vi "Config.vi"() -> ()   [LabVIEW 2020]
uses:
  Global_Variable/Global.vi
  Global_Variable/A180648.vi
  <vilib>/Utility/config.llb/NI_LVConfig.lvlib
  Libraries/S7/S7.lvlib
panel:
  in  "判定框参数":string[][](table)=[["mm"], ["KN"], ["mm"], ["KN"]]
  in  "结果判定参数":string[][](table)=[["mm"], ["KN"], ["KN"], ["KN"], [""], [""], [""], [""], [""], [""], [""], [""]]
  in  "坐标轴参数":string[][](table)=[[""], ["°/S"], ["°"], ["Nm"]]
  in  "试验项目":cluster{"拉轴":bool, "卡簧":bool}
  in  "产品型号":string(combo)
  in  "删除":bool
  in  "确定":bool
  in  "添加":bool
  in  "退出":bool
  in  "更新":bool
  # "上管柱上转向轴合成"
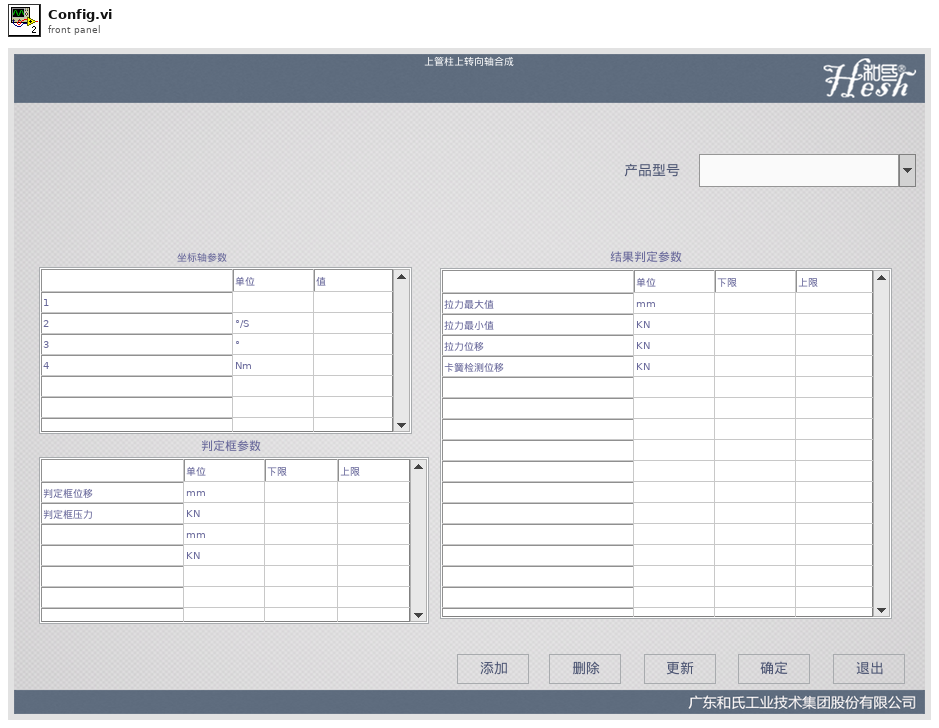
[diagram p1: front panel]
types:
  T1 = typedef "NI_LVConfig.lvlib/Config Data RefNum.ctl" = refnum<k1>
  T2 = cluster{"[0]":cluster{string, dbl, dbl}, "[1]":cluster{string, dbl, dbl}}
  T3 = cluster{"1位移":cluster{"单位":string, "下限":dbl, "上限":dbl}, "1压力":cluster{"单位":string, "下限":dbl, "上限":dbl}}
  T4 = cluster{"[0]":cluster{string, dbl, dbl}, "[1]":cluster{string, dbl, dbl}, "[2]":cluster{string, dbl, dbl}}
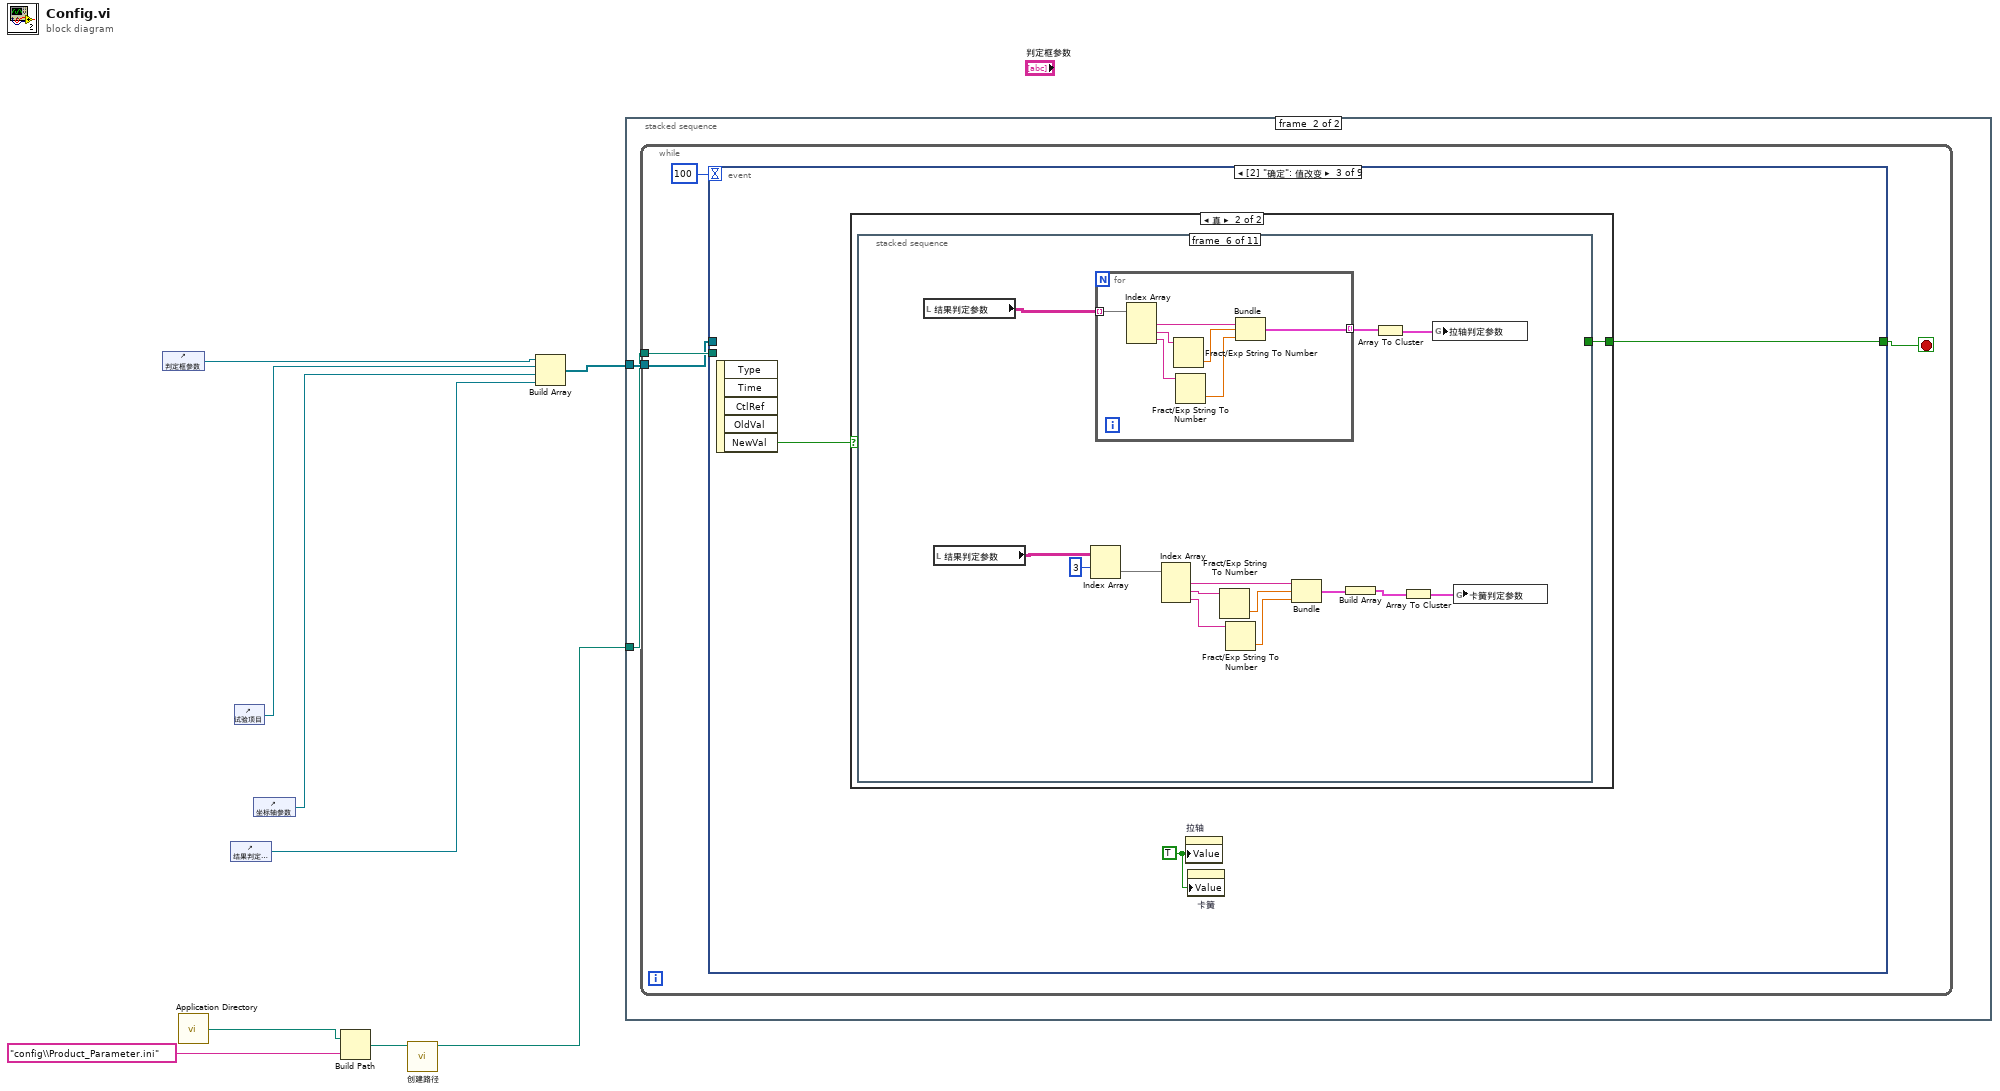
[diagram p0: block diagram]
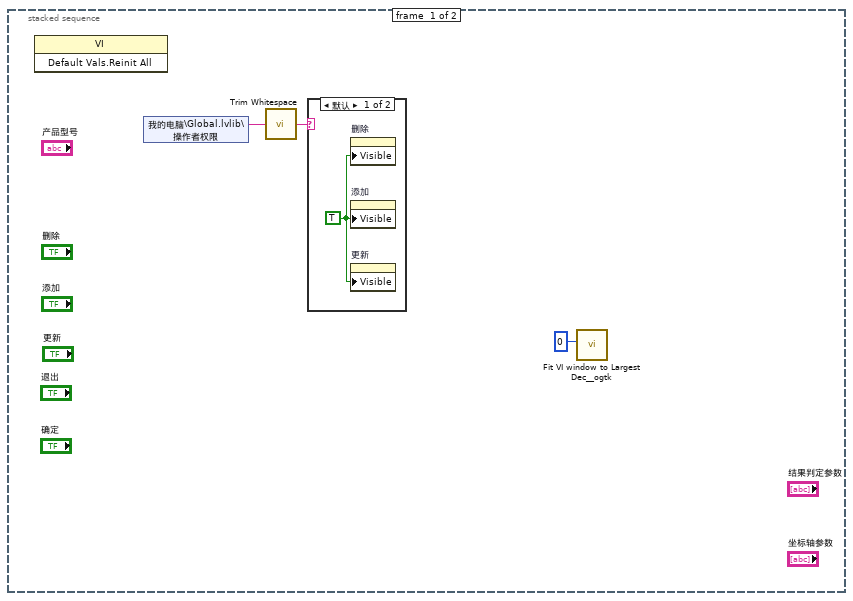
[diagram p2: hidden frame]
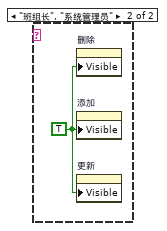
[diagram p3: hidden frame]
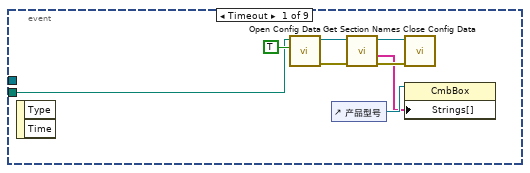
[diagram p4: hidden frame]
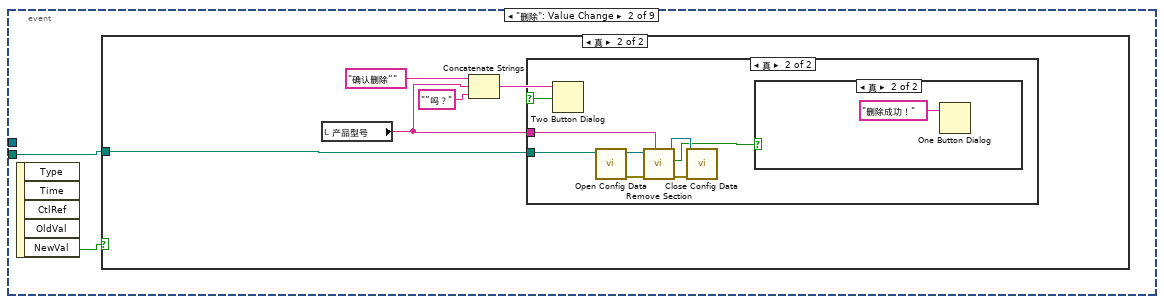
[diagram p5: hidden frame]
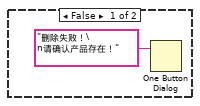
[diagram p8: hidden frame]
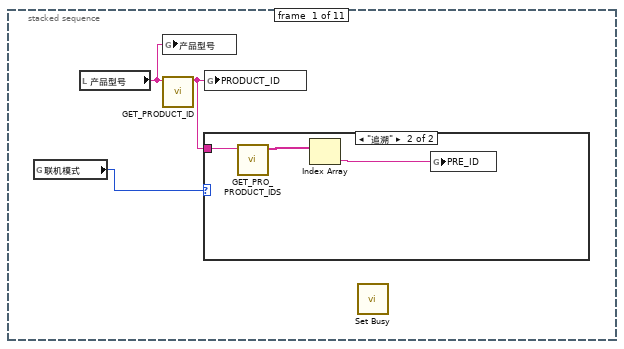
[diagram p10: hidden frame]
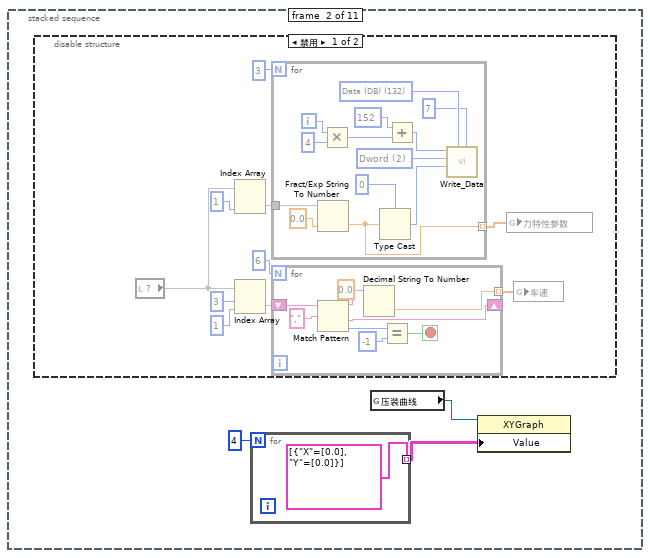
[diagram p12: hidden frame]
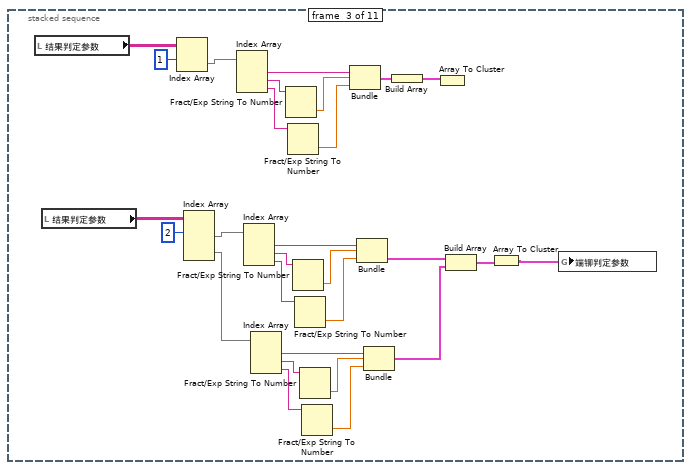
[diagram p14: hidden frame]
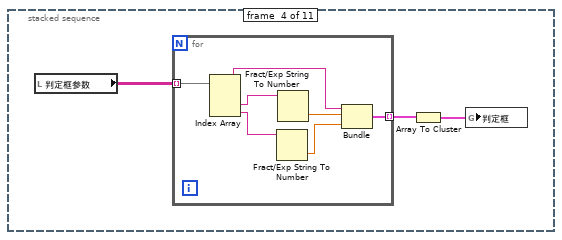
[diagram p15: hidden frame]
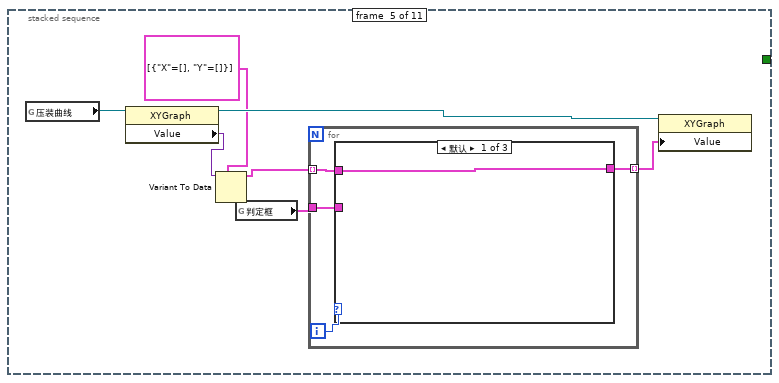
[diagram p16: hidden frame]
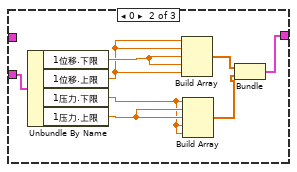
[diagram p17: hidden frame]
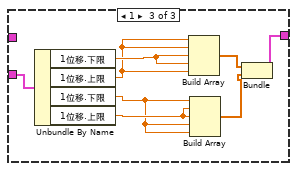
[diagram p18: hidden frame]
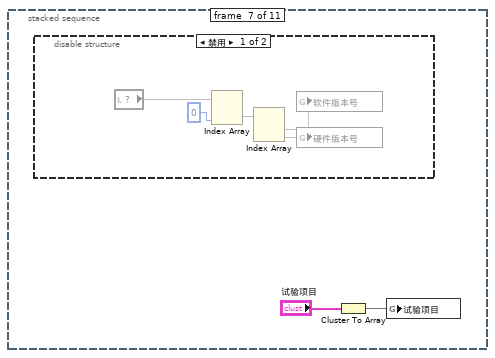
[diagram p19: hidden frame]
diagram:
  n1 = control-ref of="判定框参数"() -> (w3:refnum<vi>)
  n2 = call <vilib>:"Application Directory.vi"() -> ("Application Directory"=w8:path)
  n3 = control-ref of="结果判定参数"() -> (w7:refnum<vi>)
  n4 = control-ref of="试验项目"() -> (w2:refnum<vi>)
  n5 = control-ref of="坐标轴参数"() -> (w1:refnum<vi>)
  n6 = Build Path(base path=w8, name or relative path="config\\Product_Parameter.ini" ("名称或相对路径")) -> (appended path=w5:path)
  n7 = call "创建路径.vi"("path"=w5) -> ("path out"=w4:path)  [unwired: 9 in, 1 out]
  n8 = Build Array(w3, w2, w1, w7) -> (w9:refnum<vi>[])
  n9 = stacked-sequence {
    tunnel: w9 -> [_ w16]
    tunnel: w4 -> [_ w15]
    frame #0 {
      n10 = invoke class="VI" method="Default Vals.Reinit All"() -> ()  [unwired: 3 in, 3 out]
      n11 = shared-variable "我的电脑\\Global.lvlib\\操作者权限"() -> (w12:string)  [unwired: 1 in, 1 out]
      n12 = call <vilib>:"Trim Whitespace.vi"("string"=w12) -> ("trimmed string"=w11:string)  [unwired: 1 in]
      n13 = case shown="默认" w11 {
        frame Default {
          w13 = TRUE ("可见")
          n14 = property on="删除" class="Bool (严格)"("Visible"=w13) -> ()  [unwired: 2 in, 2 out]
          n15 = property on="添加" class="Bool (严格)"("Visible"=w13) -> ()  [unwired: 2 in, 2 out]
          n16 = property on="更新" class="Bool (严格)"("Visible"=w13) -> ()  [unwired: 2 in, 2 out]
        }
        frame "班组长", "系统管理员" {
          w14 = TRUE ("可见")
          n17 = property on="删除" class="Bool (严格)"("Visible"=w14) -> ()  [unwired: 2 in, 2 out]
          n18 = property on="添加" class="Bool (严格)"("Visible"=w14) -> ()  [unwired: 2 in, 2 out]
          n19 = property on="更新" class="Bool (严格)"("Visible"=w14) -> ()  [unwired: 2 in, 2 out]
        }
      }
      n20 = call <userlib>:"Fit VI window to Largest Dec__ogtk.vi"("border spacing (2 px)"=0) -> ()  [unwired: 5 in, 2 out]
    }
    frame #1 {
      n21 = while {
        tunnel: w15 -> [w20]
        tunnel: w16 -> [w18]
        stop <- w19 stop-if-true
        n22 = event shown="[2] \"确定\": 值改变" {
          selector: _ -> [_ _ _ _ _ _ _ _ _]
          dyn-events: _ -> [_ _ _ _ _ _ _ _ _]
          timeout: 100 -> [_ _ _ _ _ _ _ _ _]
          tunnel: w20 -> [w23 w30 _ _ w193 w220 _ w244 _]
          tunnel: [_ _ w47 _ _ _ TRUE _ TRUE] -> w19
          tunnel: w18 -> [_ _ _ _ w194 w221 _ w243 _]
          event Timeout {
            n23 = event-data() -> ()  [unwired: 1 in, 2 out]
            n24 = call <vilib>:"Open Config Data.vi"("create file if necessary (T)"=TRUE, "configuration file path"=w23) -> ("error out"=w25:errorcluster, "refnum"=w24:T1)  [unwired: 7 in, 1 out]
            n25 = control-ref of="产品型号"() -> (w22:refnum<vi>)
            n26 = call <vilib>:"Get Section Names.vi"("error in (no error)"=w25, "refnum"=w24) -> ("error out"=w27:errorcluster, "section names"=w21:string[], "refnum out"=w26:T1)  [unwired: 7 in]
            n27 = call <vilib>:"Close Config Data.vi"("error in (no error)"=w27, "refnum"=w26) -> ()  [unwired: 8 in, 2 out]
            n28 = property on="属性节点" class="CmbBox"(reference=w22, "Strings[]"=w21) -> ()  [unwired: 1 in, 2 out]
          }
          event "删除": Value Change {
            n29 = event-data() -> ("NewVal"=w29:bool)  [unwired: 1 in, 4 out]
            n30 = case shown="真" w29 {
              tunnel: w30 -> [_ w32]
              frame False {
              }
              frame True {
                n31 = local read "产品型号"() -> (w31:string)
                n32 = Concatenate Strings("确认删除“", w31, "”吗？") -> (w34:string)
                n33 = Two Button Dialog(message=w34) -> (T button?=w33:bool)  [unwired: 2 in]
                n34 = case shown="真" w33 {
                  tunnel: w32 -> [_ w38]
                  tunnel: w31 -> [_ w37]
                  frame False {
                  }
                  frame True {
                    n35 = call <vilib>:"Open Config Data.vi"("configuration file path"=w38) -> ("error out"=w40:errorcluster, "refnum"=w43:T1)  [unwired: 8 in, 1 out]
                    n36 = call <vilib>:"Remove Section.vi"("section"=w37, "error in (no error)"=w40, "refnum"=w43) -> ("error out"=w42:errorcluster, "section exists?"=w39:bool, "refnum out"=w41:T1)  [unwired: 6 in]
                    n37 = call <vilib>:"Close Config Data.vi"("error in (no error)"=w42, "refnum"=w41) -> ()  [unwired: 8 in, 2 out]
                    n38 = case shown="真" w39 {
                      frame False {
                        n39 = One Button Dialog(message="删除失败！\n请确认产品存在！" ("消息")) -> ()  [unwired: 1 in, 1 out]
                      }
                      frame True {
                        n40 = One Button Dialog(message="删除成功！" ("消息")) -> ()  [unwired: 1 in, 1 out]
                      }
                    }
                  }
                }
              }
            }
          }
          event "确定": Value Change {
            w46 = TRUE ("值")
            n41 = event-data() -> ("NewVal"=w48:bool)  [unwired: 1 in, 4 out]
            n42 = case shown="真" w48 {
              tunnel: [_ w49] -> w47
              frame False {
              }
              frame True {
                n43 = stacked-sequence {
                  tunnel: [_ _ _ _ _ _ _ _ _ _ TRUE] -> w49
                  frame #0 {
                    n44 = global read "Global.vi" "联机模式"() -> (w50:enum16{"单机", "追溯"})
                    n45 = local read "产品型号"() -> (w52:string)
                    n46 = global write "Global.vi" "产品型号"(w52) -> ()
                    n47 = call "GET_PRODUCT_ID.vi"("PRODFUCT_NAME"=w52) -> ("PRODUCT_ID"=w51:string)  [unwired: 10 in]
                    n48 = case shown="\"追溯\"" w50 {
                      tunnel: w51 -> [_ w55]
                      frame "单机", Default {
                      }
                      frame "追溯" {
                        n49 = call "GET_PRO_PRODUCT_IDS.vi"("PRODUCT_ID"=w55) -> ("前序工位"=w54:string[])  [unwired: 10 in]
                        n50 = Index Array(array=w54) -> (element=w53:string)  [unwired: 1 in]
                        n51 = global write "追溯Global.vi" "PRE_ID"(w53) -> ()
                      }
                    }
                    n52 = global write "追溯Global.vi" "PRODUCT_ID"(w51) -> ()
                    n53 = call <vilib>:"Set Busy.vi"() -> ()  [unwired: 10 in, 2 out]
                  }
                  frame #1 {
                    n54 = disable-structure shown="禁用" {
                      frame Disabled {
                        n55 = local read item#-1() -> (w66)
                        n56 = Index Array(array=w66, index (col)=1 ("禁用的索引 (列)")) -> (element=w69)  [unwired: 1 in]
                        n57 = Index Array(array=w66, index (row)=3 ("索引 (行)"), index (col)=1 ("禁用的索引 (列)")) -> (element=w63)
                        n58 = for {
                          N: 3 -> [_]
                          tunnel: w69 -> [w87]
                          tunnel: [w79] -> w60 mode=indexing
                          i -> [w82]
                          w89 = u16 2 items=["byte", "word", "Dword"] ("数据类型")
                          w91 = u8 132 items=["I/O (P)"=128, "Input (I)"=129, "Output (Q)"=130, "Bit Memory (M)"=131, "Data (DB)"=132, "Instance Data (DI)"=133, "Local Data (L)"=134, "Predecessor Local Data (VL)"=135] ("寄存器类型")
                          n59 = Fract/Exp String To Number(string=w87, default (0 dbl)=sgl 0.0) -> (number=w79:sgl)  [unwired: 2 in, 1 out]
                          n60 = Multiply(x=w82, y=4) -> (x*y=w83:i32)
                          n61 = Type Cast(type=u32 0 ("写入地址"), x=w79) -> (*(type *) &x=w85:u32)
                          n62 = Add(x=u32 152 ("写入地址"), y=w83) -> (x+y=w80:u32)
                          n63 = call "Write_Data.vi"("DB #"=u16 7, "寄存器类型"=w91, "写入数据"=w85, "数据类型"=w89, "写入地址"=w80) -> ()  [unwired: 4 in, 3 out]
                        }
                        n64 = for {
                          N: 6 -> [_]
                          shift-right: [w76] -> _
                          shift-left: w63 -> [w78]
                          tunnel: [w72] -> w62 mode=indexing
                          stop <- w71 stop-if-true
                          n65 = Match Pattern(string=w78, regular expression="," ("正则表达式")) -> (before substring=w73:string, after substring=w76:string, offset past match=w75:i32)  [unwired: 1 in, 1 out]
                          n66 = Decimal String To Number(string=w73, default (0L)=sgl 0.0 ("默认(0 I32)")) -> (number=w72:sgl)  [unwired: 1 in, 1 out]
                          n67 = Equal?(x=w75, y=-1) -> (x = y?=w71:bool)
                        }
                        n68 = global write "A180648.vi" "力特性参数"(w60) -> ()
                        n69 = global write "A180648.vi" "车速"(w62) -> ()
                      }
                      frame Enabled {
                      }
                    }
                    n70 = for {
                      N: 4 -> [_]
                      tunnel: [cluster{"X":dbl[], "Y":dbl[]}[] [{"X"=[0.0], "Y"=[0.0]}]] -> w58 mode=indexing
                    }
                    n71 = global read "A180648.vi" "压装曲线"() -> (w56:refnum<vi>)
                    n72 = property class="XYGraph"(reference=w56, "Value"=w58) -> ()  [unwired: 1 in, 2 out]
                  }
                  frame #2 {
                    n73 = local read "结果判定参数"() -> (w113:string[][])
                    n74 = local read "结果判定参数"() -> (w106:string[][])
                    n75 = Index Array(array=w113, index (row)=1 ("索引 (行)")) -> (element=w119:string[])  [unwired: 1 in]
                    n76 = Index Array(array=w106, index (row) #1=2 ("索引 (行)")) -> (element #1=w100:string[], element #2=w94:string[])  [unwired: 3 in]
                    n77 = Index Array(array=w119) -> (element #1=w118:string, element #2=w117:string, element #3=w115:string)  [unwired: 3 in]
                    n78 = Index Array(array=w100) -> (element #1=w101:string, element #2=w102:string, element #3=w104:string)  [unwired: 3 in]
                    n79 = Index Array(array=w94) -> (element #1=w99:string, element #2=w98:string, element #3=w96:string)  [unwired: 3 in]
                    n80 = Fract/Exp String To Number(string=w117) -> (number=w116:dbl)  [unwired: 3 in, 1 out]
                    n81 = Fract/Exp String To Number(string=w115) -> (number=w114:dbl)  [unwired: 3 in, 1 out]
                    n82 = Fract/Exp String To Number(string=w102) -> (number=w103:dbl)  [unwired: 3 in, 1 out]
                    n83 = Fract/Exp String To Number(string=w104) -> (number=w105:dbl)  [unwired: 3 in, 1 out]
                    n84 = Fract/Exp String To Number(string=w98) -> (number=w97:dbl)  [unwired: 3 in, 1 out]
                    n85 = Fract/Exp String To Number(string=w96) -> (number=w95:dbl)  [unwired: 3 in, 1 out]
                    n86 = Bundle(w118, w116, w114) -> (w111:cluster{string, dbl, dbl})  [unwired: 1 in]
                    n87 = Bundle(w101, w103, w105) -> (w108:cluster{string, dbl, dbl})  [unwired: 1 in]
                    n88 = Bundle(w99, w97, w95) -> (w93:cluster{string, dbl, dbl})  [unwired: 1 in]
                    n89 = Build Array(w111) -> (w110:cluster{string, dbl, dbl}[])
                    n90 = Array To Cluster(array=w110) -> ()  [unwired: 1 out]
                    n91 = Build Array(w108, w93) -> (w109:cluster{string, dbl, dbl}[])
                    n92 = Array To Cluster(array=w109) -> (cluster=w92:T2)
                    n93 = global write "判定参数.vi" "端铆判定参数"(w92) -> ()
                  }
                  frame #3 {
                    n94 = local read "判定框参数"() -> (w122:string[][])
                    n95 = for {
                      tunnel: w122 -> [w129] mode=indexing
                      tunnel: [w123] -> w121 mode=indexing
                      n96 = Index Array(array=w129) -> (element #1=w126:string, element #2=w128:string, element #3=w127:string)  [unwired: 3 in]
                      n97 = Fract/Exp String To Number(string=w127) -> (number=w124:dbl)  [unwired: 3 in, 1 out]
                      n98 = Fract/Exp String To Number(string=w128) -> (number=w125:dbl)  [unwired: 3 in, 1 out]
                      n99 = Bundle(w126, w125, w124) -> (w123:cluster{string, dbl, dbl})  [unwired: 1 in]
                    }
                    n100 = Array To Cluster(array=w121) -> (cluster=w120:T2)
                    n101 = global write "判定参数.vi" "判定框"(w120) -> ()
                  }
                  frame #4 {
                    n102 = global read "A180648.vi" "压装曲线"() -> (w136:refnum<vi>)
                    n103 = property class="XYGraph"(reference=w136) -> (reference out=w133:refnum<vi>, "Value"=w135:variant)  [unwired: 1 in, 1 out]
                    n104 = Variant To Data(type=cluster{"X":dbl[], "Y":dbl[]}[] [{"X"=[], "Y"=[]}], Variant=w135) -> (data=w134:cluster{"X":dbl[], "Y":dbl[]}[])  [unwired: 1 in, 1 out]
                    n105 = global read "判定参数.vi" "判定框"() -> (w130:T3)
                    n106 = for {
                      tunnel: w134 -> [w139] mode=indexing
                      tunnel: [w138] -> w131 mode=indexing
                      tunnel: w130 -> [w137]
                      i -> [w140]
                      n107 = case shown="默认" w140 {
                        tunnel: w139 -> [w141 _ _]
                        tunnel: [w141 w144 w152] -> w138
                        tunnel: w137 -> [_ w149 w153]
                        frame Default {
                        }
                        frame 0 {
                          n108 = Unbundle By Name(w149) -> ("1位移.下限"=w148:dbl, "1位移.上限"=w147:dbl, "1压力.下限"=w142:dbl, "1压力.上限"=w143:dbl)
                          n109 = Build Array(w147, w147, w148, w148, w147) -> (w146:dbl[])
                          n110 = Build Array(w142, w143, w143, w142, w142) -> (w145:dbl[])
                          n111 = Bundle(w146, w145) -> (w144:cluster{dbl[], dbl[]})  [unwired: 1 in]
                        }
                        frame 1 {
                          n112 = Unbundle By Name(w153) -> ("1位移.下限"=w157:dbl, "1位移.上限"=w156:dbl, "1位移.下限"=w150:dbl, "1位移.上限"=w151:dbl)
                          n113 = Build Array(w156, w156, w157, w157, w156) -> (w155:dbl[])
                          n114 = Build Array(w150, w151, w151, w150, w150) -> (w154:dbl[])
                          n115 = Bundle(w155, w154) -> (w152:cluster{dbl[], dbl[]})  [unwired: 1 in]
                        }
                      }
                    }
                    n116 = property class="XYGraph"(reference=w133, "Value"=w131) -> ()  [unwired: 1 in, 2 out]
                  }
                  frame #5 {
                    n117 = local read "结果判定参数"() -> (w171:string[][])
                    n118 = local read "结果判定参数"() -> (w168:string[][])
                    n119 = Index Array(array=w168, index (row)=3 ("索引 (行)")) -> (element=w166:string[])  [unwired: 1 in]
                    n120 = for {
                      tunnel: w171 -> [w173] mode=indexing
                      tunnel: [w172] -> w169 mode=indexing
                      n121 = Index Array(array=w173) -> (element #1=w178:string, element #2=w177:string, element #3=w175:string)  [unwired: 3 in]
                      n122 = Fract/Exp String To Number(string=w177) -> (number=w176:dbl)  [unwired: 3 in, 1 out]
                      n123 = Fract/Exp String To Number(string=w175) -> (number=w174:dbl)  [unwired: 3 in, 1 out]
                      n124 = Bundle(w178, w176, w174) -> (w172:cluster{string, dbl, dbl})  [unwired: 1 in]
                    }
                    n125 = Index Array(array=w166) -> (element #1=w165:string, element #2=w164:string, element #3=w162:string)  [unwired: 3 in]
                    n126 = Fract/Exp String To Number(string=w164) -> (number=w163:dbl)  [unwired: 3 in, 1 out]
                    n127 = Fract/Exp String To Number(string=w162) -> (number=w161:dbl)  [unwired: 3 in, 1 out]
                    n128 = Bundle(w165, w163, w161) -> (w160:cluster{string, dbl, dbl})  [unwired: 1 in]
                    n129 = Build Array(w160) -> (w159:cluster{string, dbl, dbl}[])
                    n130 = Array To Cluster(array=w169) -> (cluster=w170:T4)
                    n131 = Array To Cluster(array=w159) -> (cluster=w158:cluster{"[0]":cluster{string, dbl, dbl}})
                    n132 = global write "判定参数.vi" "拉轴判定参数"(w170) -> ()
                    n133 = global write "判定参数.vi" "卡簧判定参数"(w158) -> ()
                  }
                  frame #6 {
                    n134 = disable-structure shown="禁用" {
                      frame Disabled {
                        n135 = local read item#-1() -> (w185)
                        n136 = Index Array(array=w185, index (col)=0 ("禁用的索引 (列)")) -> (element=w183)  [unwired: 1 in]
                        n137 = Index Array(array=w183) -> (element #1=w182, element #2=w181)  [unwired: 2 in]
                        n138 = global write "Global.vi" "软件版本号"(w182) -> ()
                        n139 = global write "Global.vi" "硬件版本号"(w181) -> ()
                      }
                      frame Enabled {
                      }
                    }
                    n140 = Cluster To Array(cluster="试验项目") -> (array=w180:bool[])
                    n141 = global write "Global.vi" "试验项目"(w180) -> ()
                  }
                  frame #7 {
                    n142 = call <vilib>:"Unset Busy.vi"() -> ()  [unwired: 11 in, 1 out]
                  }
                  frame #8 {
                    n143 = global read "Global.vi" "更换产品"() -> (w187:refnum<vi>)
                    n144 = vi-ref "Auto.vi"() -> (w186:refnum<vi>)
                    n145 = property class="VIRef"(reference=w187, "Val(Sgnl)"=w186) -> ()  [unwired: 1 in, 2 out]
                  }
                  frame #9 {
                    w188 = "参数装载成功！" ("消息")
                    n146 = call "浮动通知.vi"("通知内容"=w188) -> ()  [unwired: 11 in]
                    n147 = One Button Dialog(message=w188) -> ()  [unwired: 1 in, 1 out]
                  }
                  frame #10 {
                    n148 = control-ref of="本VI"() -> (w189:refnum<vi>)
                    n149 = invoke class="VI" method="FP.Close"(reference=w189) -> ()  [unwired: 2 in, 3 out]
                  }
                }
              }
            }
            n150 = property on="拉轴" class="Bool (严格)"("Value"=w46) -> ()  [unwired: 2 in, 2 out]
            n151 = property on="卡簧" class="Bool (严格)"("Value"=w46) -> ()  [unwired: 2 in, 2 out]
          }
          event "试验项目.卡簧": Value Change {
            n152 = event-data() -> ("NewVal"=w191:bool)  [unwired: 1 in, 5 out]
            n153 = case shown="真" w191 {
              frame False {
              }
              frame True {
                (unwired) FALSE ("值")
              }
            }
          }
          event "添加": Value Change {
            n154 = event-data() -> ("NewVal"=w192:bool)  [unwired: 1 in, 4 out]
            n155 = case shown="真" w192 {
              tunnel: w194 -> [_ w198]
              tunnel: w193 -> [_ w197]
              frame False {
              }
              frame True {
                n156 = call "产品添加提示：用户输入"() -> ("产品型号"=w195:string, "确定"=w196:bool)  [unwired: 17 in, 1 out]
                n157 = case shown="真" w196 {
                  tunnel: w198 -> [_ w201]
                  tunnel: w197 -> [_ w200]
                  tunnel: w195 -> [_ w199]
                  frame False {
                  }
                  frame True {
                    n158 = case shown="默认" w199 {
                      selector: w199 -> [_ w204]
                      tunnel: w201 -> [_ w207]
                      tunnel: w200 -> [_ w206]
                      frame "" {
                        n159 = One Button Dialog(message="产品名称不得为空!" ("text")) -> ()  [unwired: 1 in, 1 out]
                      }
                      frame Default {
                        n160 = property on="产品型号" class="CmbBox"() -> ("Strings[]"=w205:string[])  [unwired: 2 in, 2 out]
                        n161 = Search 1D Array(1D array=w205, element=w204) -> (index of element=w203:i32)  [unwired: 1 in]
                        n162 = case shown="-1" w203 {
                          tunnel: w207 -> [_ w211]
                          tunnel: w206 -> [_ w210]
                          tunnel: w204 -> [_ w209]
                          frame Default {
                            n163 = One Button Dialog(message="产品已存在！" ("消息")) -> ()  [unwired: 1 in, 1 out]
                          }
                          frame -1 {
                            n164 = stacked-sequence {
                              tunnel: w211 -> [w217 _]
                              tunnel: w210 -> [w216 _]
                              tunnel: w209 -> [w215 _]
                              frame #0 {
                                n165 = call <vilib>:"Set Busy.vi"() -> ("error out"=w213:errorcluster)  [unwired: 10 in, 1 out]
                                n166 = call "Read_Write INI File.vi"("Mode"=enum16{"Read", "Write"}."Write", "Section"=w215, "error in"=w213, "Filepath"=w216, "Ctl Refnum"=w217) -> ("error out"=w212:errorcluster)  [unwired: 6 in]
                                n167 = call <vilib>:"Unset Busy.vi"("error in (no error)"=w212) -> ()  [unwired: 10 in, 1 out]
                              }
                              frame #1 {
                                n168 = One Button Dialog(message="添加成功！" ("消息")) -> ()  [unwired: 1 in, 1 out]
                              }
                            }
                          }
                        }
                      }
                    }
                  }
                }
              }
            }
          }
          event "产品型号": Value Change {
            n169 = event-data() -> ("NewVal"=w219:string)  [unwired: 1 in, 4 out]
            n170 = stacked-sequence {
              tunnel: w221 -> [_ _ w225]
              tunnel: w220 -> [_ _ w224]
              tunnel: w219 -> [_ w223 _]
              frame #0 {
                n171 = control-ref of="本VI"() -> (w222:refnum<vi>)
                n172 = invoke class="VI" method="Default Vals.Reinit All"(reference=w222) -> ()  [unwired: 2 in, 3 out]
              }
              frame #1 {
                n173 = local write "产品型号"(w223) -> ()
              }
              frame #2 {
                n174 = disable-structure shown="启用" {
                  disable-tunnel: w225 -> [w227 w236]
                  disable-tunnel: w224 -> [w226 w237]
                  frame Disabled {
                    n175 = for {
                      tunnel: w227 -> [w230] mode=indexing
                      tunnel: w226 -> [w229]
                      n176 = local read "产品型号"() -> (w228:string)
                      n177 = call "Read_Write ParaINI File.vi"("Mode"=enum16{"Read", "Write"}."Read", "Section"=w228, "Filepath"=w229, "Ctl Refnum"=w230) -> ()  [unwired: 7 in, 1 out]
                    }
                  }
                  frame Enabled {
                    n178 = call <vilib>:"Set Busy.vi"() -> ("error out"=w232:errorcluster)  [unwired: 10 in, 1 out]
                    n179 = local read "产品型号"() -> (w235:string)
                    n180 = call "Read_Write INI File.vi"("Mode"=enum16{"Read", "Write"}."Read", "Section"=w235, "error in"=w232, "Filepath"=w237, "Ctl Refnum"=w236) -> ("error out"=w233:errorcluster)  [unwired: 6 in]
                    n181 = call <vilib>:"Unset Busy.vi"("error in (no error)"=w233) -> ()  [unwired: 10 in, 1 out]
                  }
                }
              }
            }
          }
          event "退出": Value Change {
            n182 = event-data() -> ()  [unwired: 1 in, 5 out]
            n183 = control-ref of="本VI"() -> (w240:refnum<vi>)
            n184 = invoke class="VI" method="FP.Close"(reference=w240) -> (reference out=w238:refnum<vi>, error out=w239:errorcluster)  [unwired: 2 in, 1 out]
            n185 = Close Reference(reference=w238, error in (no error)=w239) -> ()  [unwired: 1 out]
          }
          event "更新": Value Change {
            n186 = event-data() -> ("NewVal"=w242:bool)  [unwired: 1 in, 4 out]
            n187 = case shown="真" w242 {
              tunnel: w244 -> [_ w247]
              tunnel: w243 -> [_ w246]
              frame False {
              }
              frame True {
                n188 = disable-structure shown="启用" {
                  disable-tunnel: w247 -> [w250 w261]
                  disable-tunnel: w246 -> [w249 w256]
                  disable-tunnel: [w248 w258] -> w245
                  frame Disabled {
                    n189 = for {
                      tunnel: w250 -> [w253]
                      tunnel: w249 -> [w252] mode=indexing
                      tunnel: [w251] -> w248
                      n190 = local read "产品型号"() -> (w255:string)
                      n191 = call "Read_Write ParaINI File.vi"("Mode"=enum16{"Read", "Write"}."Write", "Section"=w255, "Filepath"=w253, "Ctl Refnum"=w252) -> ("error out"=w251:errorcluster)  [unwired: 7 in]
                    }
                  }
                  frame Enabled {
                    n192 = call <vilib>:"Set Busy.vi"() -> ("error out"=w257:errorcluster)  [unwired: 10 in, 1 out]
                    n193 = local read "产品型号"() -> (w260:string)
                    n194 = call "Read_Write INI File.vi"("Mode"=enum16{"Read", "Write"}."Write", "Section"=w260, "error in"=w257, "Filepath"=w261, "Ctl Refnum"=w256) -> ("error out"=w258:errorcluster)  [unwired: 6 in]
                  }
                }
                n195 = case shown="无错误" w245 {
                  frame No Error {
                    n196 = call <vilib>:"Unset Busy.vi"() -> ()  [unwired: 11 in, 1 out]
                    n197 = Wait (ms)(milliseconds to wait=u32 500 ("等待时间（毫秒）")) -> ()  [unwired: 1 out]
                    n198 = One Button Dialog(message="更新成功！" ("通知内容")) -> ()  [unwired: 1 in, 1 out]
                  }
                  frame Error {
                    n199 = Wait (ms)(milliseconds to wait=u32 500 ("等待时间（毫秒）")) -> ()  [unwired: 1 out]
                    n200 = call "浮动通知.vi"("通知内容"="更新失败！") -> ()  [unwired: 11 in]
                  }
                }
              }
            }
          }
          event Panel Close {
            n201 = event-data() -> ()  [unwired: 1 in, 3 out]
          }
        }
      }
    }
  }
